vi "Set Caption.vi"(8 "error in":errorcluster, 11 "DIG_IO in":refnum<class "DIG_IO.lvclass">) -> (0 "error out":errorcluster, 3 "DIG_IO out":refnum<class "DIG_IO.lvclass">)   [LabVIEW 2019, in "DIG_IO.lvlib" / "DIG_IO.lvclass"]
uses:
  Library/DIG_IO.lvclass
  Library/DIG_IO.lvclass/DIG_IO.ctl
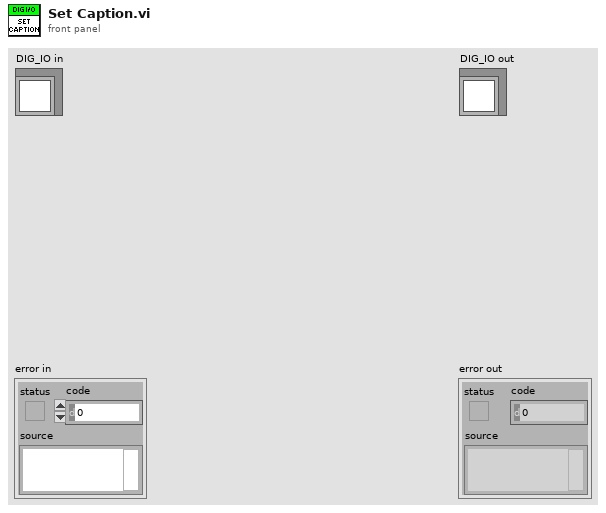
[diagram p1: front panel]
types:
  T1 = enum8{"Enabled", "Disabled", "Disabled and Grayed Out"}[]
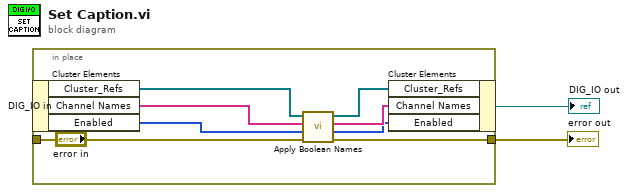
[diagram p0: block diagram]
diagram:
  n1 = in-place {
    in-place-border: "error in" -> [w8]
    in-place-border: [w7] -> w1
    n2 = in-place-cluster #1("DIG_IO in") -> ("Cluster_Refs"=w12:refnum<vi>[], "Channel Names"=w11:string[], "Enabled"=w6:T1)
    n3 = call "Apply Boolean Names.vi"("error in"=w8, "Enabled In"=w6, "Names in"=w11, "Cluster_Refs in"=w12) -> ("error out"=w7:errorcluster, "Enabled out"=w5:T1, "Names out"=w9:string[], "Cluster_Refs Out"=w10:refnum<vi>[])  [unwired: 4 in]
    n4 = in-place-cluster #1("Cluster_Refs"=w10, "Channel Names"=w9, "Enabled"=w5) -> (→"DIG_IO out":refnum<class "DIG_IO.lvclass">)
  }
  "error out" <- w1
